vi "TcpServer_Init.vi"(10 "local port":u16, 11 "response event":T2) -> (1 "Message queue":T1, 3 "TcpServerDriver":refnum<class "TcpServerDriver.lvclass">)   [LabVIEW 2013, in "TcpServerDriver.lvclass"]
uses:
  TcpServerDriver.lvclass
  response_event.ctl
  response.ctl
  driver_status.ctl
  message_queue.ctl
  Message/BaseMessage/BaseMessage.lvclass
  Message/MixerMessage/MixerMessage.lvclass
  Reader/TcpServer/TcpServer.lvclass
  BaseDriver/Write Notify idle.vi
  BaseDriver/Write Idle read.vi
  BaseDriver/Write Poll interval.vi
  BaseDriver/Write Reader.vi
  BaseDriver/Write Wait for response.vi
  BaseDriver/Write Reconnect.vi
  BaseDriver/BaseDriver.lvclass
  TcpDriver/TcpDriver.lvclass
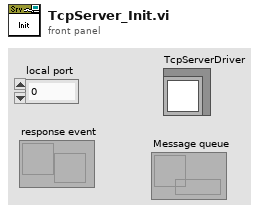
[diagram p1: front panel]
types:
  T1 = typedef "message_queue.ctl" = refnum<queue>
  T2 = typedef "response_event.ctl" = refnum<user-event>
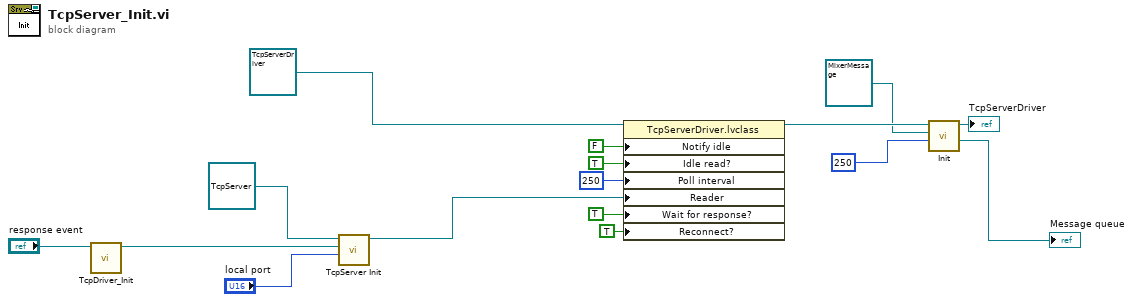
[diagram p0: block diagram]
diagram:
  n1 = call "TcpDriver_Init.vi"("response event"="response event") -> ("TcpDriver out"=w3:refnum<class "TcpDriver.lvclass">)  [unwired: 9 in, 1 out]
  n2 = call "TcpServer Init.vi"("local port"="local port", "Driver to run"=w3, "TcpServer in"=refnum<class "TcpServer.lvclass"> refnum) -> ("TcpServer out"=w6:refnum<class "TcpServer.lvclass">)  [unwired: 7 in, 1 out]
  n3 = property class="TcpServerDriver.lvclass"(reference=refnum<class "TcpServerDriver.lvclass"> refnum ("TcpServerDriver.lvclass"), "Notify idle"=FALSE, "Idle read?"=TRUE, "Poll interval"=250, "Reader"=w6, "Wait for response?"=TRUE, "Reconnect?"=TRUE) -> (reference out=w12:refnum<class "TcpServerDriver.lvclass">)  [unwired: 1 in, 1 out]
  n4 = call "Init.vi"("Poll interval"=250, "Message type"=refnum<class "MixerMessage.lvclass"> refnum ("MixerMessage.lvclass"), "BaseDriver in"=w12) -> ("Message queue"=→"Message queue":T1, "BaseDriver out"=→"TcpServerDriver":refnum<class "TcpServerDriver.lvclass">)  [unwired: 6 in, 1 out]
